vi "Configure Sparse Marker [SM] Core.vi"(5 "Destination Terminal (None)":string(combo) caption="destination terminal (None)", 6 "Indexes Array":i64[](array[numeric]) caption="indexes array", 7 "Number Indexes":i64 caption="number indexes" format="%.0g", 8 "error in (no error)":errorcluster, 9 "Waveform Handle":i32 caption="waveform handle" format="%.0g", 10 "Marker Name (\"\")":string caption="marker name (\"\")", 11 "IVI_Fgen in":refnum<class "IVI_Fgen.lvclass">) -> (0 "error out":errorcluster, 3 "IVI_Fgen out":refnum<class "IVI_Fgen.lvclass">)   [LabVIEW 2013, in "IVI_Fgen.lvlib" / "IVI_Fgen.lvclass"]
doc: "This VI configures the common sparse marker properties. These properties are the sparse marker waveform handle and destination.\n \nThis VI also configures which waveform and sample number the output is associated with.\n\nNote:\n\n(1) This VI is part of the IviFgenSparseMarker [SM] extension group."
uses:
  IVI_Fgen.lvclass
  IVI_Fgen.lvclass/IVI_Fgen.ctl
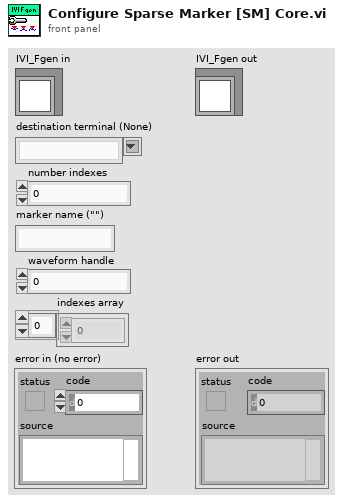
[diagram p1: front panel]
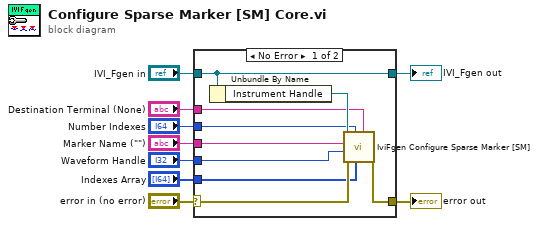
[diagram p0: block diagram]
diagram:
  n1 = case shown="No Error" "error in (no error)" {
    selector: "error in (no error)" -> [w16 w20]
    tunnel: [w15 w20] -> w8
    tunnel: [w18 w19] -> w6
    tunnel: "IVI_Fgen in" -> [w18 w19]
    tunnel: "Marker Name (\"\")" -> [w14 _]
    tunnel: "Destination Terminal (None)" -> [w13 _]
    tunnel: "Number Indexes" -> [w12 _]
    tunnel: "Waveform Handle" -> [w11 _]
    tunnel: "Indexes Array" -> [w10 _]
    frame No Error {
      n2 = Unbundle By Name(w18) -> ("Instrument Handle"=w17:refnum<k15>)
      n3 = call <vilib>:"IviFgen Configure Sparse Marker [SM].vi"("Destination Terminal (None)"=w13, "Indexes Array"=w10, "Number Indexes"=w12, "error in (no error)"=w16, "Waveform Handle"=w11, "Marker Name (\"\")"=w14, "instrument handle"=w17) -> ("error out"=w15:errorcluster)  [unwired: 3 in, 1 out]
    }
    frame Error {
    }
  }
  "error out" <- w8
  "IVI_Fgen out" <- w6
